vi "PCO_GetBufferStatusWaitforimage.vi"(3 "error in":errorcluster, 4 "expected seconds":dbl=0.01, 5 "sBufNr":i16, 6 "Handle":u64) -> (0 "error out":errorcluster {"code" items=["no error"=0, "init failed"=-1, "timeout in anx function"=-2, "function call with wrong parameter"=-3, "cannot locate PCI card or driver"=-4, "cannot allocate DMA buffer"=-5, "reserved (no init?)"=-6, "DMA timeout"=-7, "invalid camera mode"=-8, "no driver installed"=-9, "no PCI biso found"=-10, "device is hold by another process"=-11, "error reading or writing data to board"=-12, "wrong driver function"=-13, "reserved"=-14, "reserved"=-15, "reserved"=-16, "reserved"=-17, "reserved"=-18, "reserved"=-19, "LOAD_COC error (program memory)"=-20, "too many COC values"=-21, "CCD/electronics temperatue out of range"=-22, "buffer allocate error"=-23, "READ_Image reeor"=-24, "set/reset buffer flags failed"=-25, "buffer is used"=-26, "call to a windows function failed"=-27, "DMA error"=-28, "cannot open file"=-29, "registry error"=-30, "open dialog error"=-31, "need newer called vxd or dll"=-32, "Warning no image in buffer"=100, "Warning: too dark"=101, "Warning: too bright"=102, "Warning: 1 or 2 values changed"=103, "Werning: buffer for sting too short"=104]}, 2 "Handle Out":u64)   [LabVIEW 2011]
panel:
  out "Numeric":i32
  # "first wait 96%\nthen repeated wait with 5%"
  # "110: wait while\ncoc is running (bit2)\nno data available (bit1)"
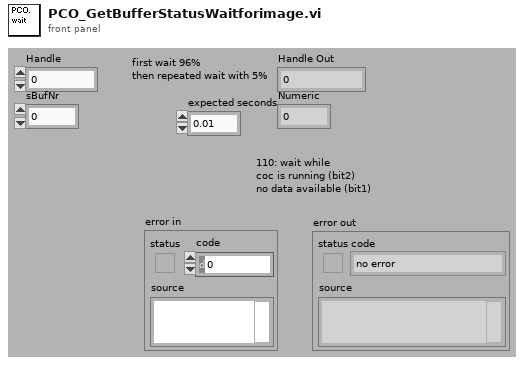
[diagram p1: front panel]
types:
  T1 = cluster{"allocated":bool, "event inside DLL":bool, "allocated externally":bool, "event set":bool}
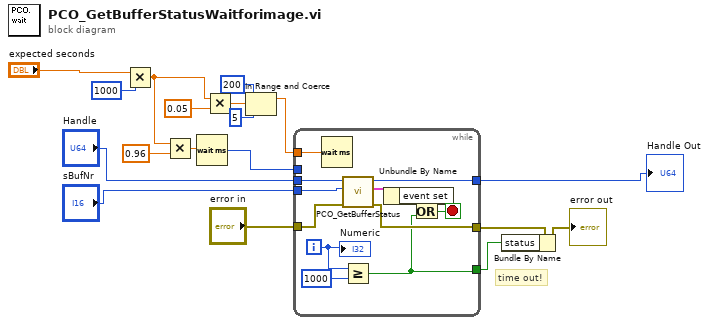
[diagram p0: block diagram]
diagram:
  # "time out!"
  n1 = Multiply(x="expected seconds", y=u32 1000) -> (x*y=w4:dbl)
  n2 = Multiply(x=w4, y=0.96) -> (x*y=w16:dbl)
  n3 = Wait (ms)(milliseconds to wait=w16) -> (millisecond timer value=w8:u32)
  n4 = Multiply(x=w4, y=0.05) -> (x*y=w13:dbl)
  n5 = In Range and Coerce(upper limit=200, x=w13, lower limit=5) -> (coerced(x)=w9:dbl)  [unwired: 1 out]
  n6 = while {
    tunnel: "error in" -> [w27]
    tunnel: [w26] -> w17
    tunnel: w9 -> [w30]
    tunnel: w8 -> [_]
    tunnel: "Handle" -> [w25]
    tunnel: [w24] -> w6
    tunnel: "sBufNr" -> [w23]
    tunnel: [w19] -> w1
    i -> [w22]
    stop <- w20 stop-if-true
    n7 = Wait (ms)(milliseconds to wait=w30) -> ()  [unwired: 1 out]
    n8 = call "PCO_GetBufferStatus.vi"("error in (no error)"=w27, "sBufNr"=w23, "Handle"=w25) -> ("error out"=w26:errorcluster, "StatusDll"=w29:T1, "Handle Out"=w24:u64)  [unwired: 6 out]
    n9 = Greater Or Equal?(x=w22, y=1000) -> (x >= y?=w19:bool)
    n10 = Unbundle By Name(w29) -> ("event set"=w28:bool)
    n11 = Or(x=w28, y=w19) -> (x .or. y?=w20:bool)
    "Numeric" <- w22
  }
  "Handle Out" <- w6
  n12 = Bundle By Name(cluster=w17, "status"=w1) -> (→"error out":errorcluster)
